vi "Dock or Undock.vi"(8 "error in (no error)":errorcluster, 10 "Action":T1, 11 "Assert Startup UI in":refnum<class "Assert Startup UI.lvclass">) -> (0 "error out":errorcluster, 3 "Assert Startup UI out":refnum<class "Assert Startup UI.lvclass">)   [LabVIEW 2016, in "Assert API Components.lvlib" / "Assert Startup UI.lvlib" / "Assert Startup UI.lvclass"]
uses:
  Assert Startup UI.lvclass
  System Tray Docking Actions.ctl
  Assert Startup UI.lvclass/Assert Startup UI.ctl
  System Tray/NotifyIcon.lvclass
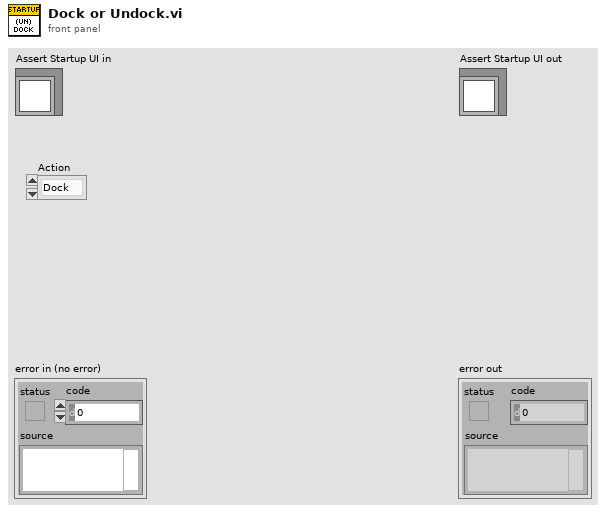
[diagram p1: front panel]
types:
  T1 = typedef "Assert API Components.lvlib/Assert Startup UI.lvlib/Assert Startup UI.lvclass/System Tray Docking Actions.ctl" = enum16{"Dock", "Undock"}
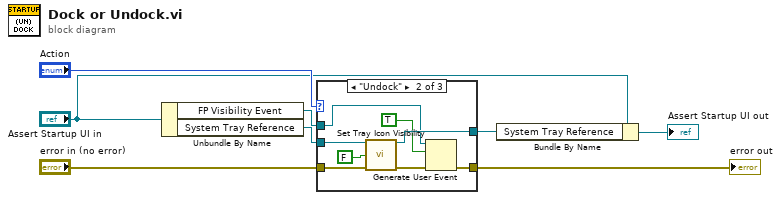
[diagram p0: block diagram]
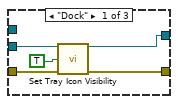
[diagram p2: hidden frame]
diagram:
  n1 = Unbundle By Name("Assert Startup UI in") -> ("FP Visibility Event"=w1:refnum<user-event>, "System Tray Reference"=w6:refnum<class "NotifyIcon.lvclass">)
  n2 = case shown="\"Undock\"" "Action" {
    tunnel: w6 -> [w13 w21 w23]
    tunnel: [w12 w20 w23] -> w4
    tunnel: "error in (no error)" -> [w11 w19 w22]
    tunnel: [w10 w16 w22] -> w2
    tunnel: w1 -> [_ w15 _]
    frame "Dock" {
      n3 = call "Set Tray Icon Visibility.vi"("NotifyIcon in"=w13, "Show Tray Icon"=TRUE, "error in (no error)"=w11) -> ("NotifyIcon out"=w12:refnum<class "NotifyIcon.lvclass">, "error out"=w10:errorcluster)  [unwired: 11 out]
    }
    frame "Undock" {
      n4 = call "Set Tray Icon Visibility.vi"("NotifyIcon in"=w21, "Show Tray Icon"=FALSE, "error in (no error)"=w19) -> ("NotifyIcon out"=w20:refnum<class "NotifyIcon.lvclass">, "error out"=w18:errorcluster)  [unwired: 11 out]
      n5 = Generate User Event(user event=w15, event data cluster=TRUE ("event data"), error in=w18) -> (error out=w16:errorcluster)  [unwired: 1 in, 1 out]
    }
    frame Default {
    }
  }
  "error out" <- w2
  n6 = Bundle By Name(cluster="Assert Startup UI in", "System Tray Reference"=w4) -> (→"Assert Startup UI out":refnum<class "Assert Startup UI.lvclass">)
